vi "fgt get pressure Channel Count.vi"(8 "error in (no error)":errorcluster) -> (0 "error out":errorcluster, 3 "nbPChan out":u32)   [LabVIEW 2020, in "fgt_SDK.lvlib"]
doc: "Get total number of initialized pressure channels. It is the sum of all MFCS, MFCS-EZ and FlowEZ pressure controllers"
uses:
  fgt_SDK.lvlib
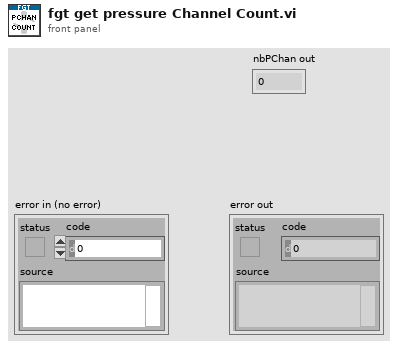
[diagram p1: front panel]
types:
  T1 = typedef "fgt_SDK.lvlib/fgt_STATUS_INFO.ctl" = cluster{"InstrType":T2, "instrSN":u16, "errorCode":u8, "infoCode":u8, "detail":string}
  T2 = typedef "fgt_SDK.lvlib/fgt_INSTRUMENT_TYPE.ctl" = enum32{"None", "MFCS", "MFCS_EZ", "FRP", "LineUP", "IPS"}
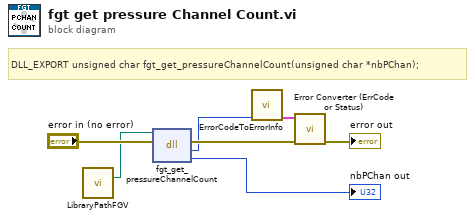
[diagram p0: block diagram]
diagram:
  # "DLL_EXPORT unsigned char fgt_get_pressureChannelCount(unsigned char *nbPChan);"
  n1 = call "LibraryPathFGV.vi"() -> ("Path Out"=w1:path)  [unwired: 14 in, 1 out]
  n2 = dll-call lib="C:/Workspace/fgt-SDK/LabVIEW/dlls/fgt_SDK_*.*" fn="fgt_get_pressureChannelCount"(path in=w1, error in="error in (no error)") -> (error out=w6:errorcluster, "return type"=w3:u8, "nbPChan"=→"nbPChan out":u8)  [unwired: 2 in, 1 out]
  n3 = call "ErrorCodeToErrorInfo.vi"("return type"=w3) -> ("StatusInfo"=w4:T1)  [unwired: 10 in]
  n4 = call "Error Converter (ErrCode or Status).vi"("error in (no error)"=w6, "StatusInfo"=w4) -> ("error out"=→"error out":errorcluster)  [unwired: 9 in]
